vi "AK Aktion Name.vi"(11 "Aktionen":T1) -> (3 "Aktions Name":string)   [LabVIEW 2020, in "AK-Schnittstelle.lvlib"]
uses:
  AK-Schnittstelle.lvlib
  Aktionen AK.ctl
  <vilib>/Utility/Data Type/NI_Data Type.lvlib
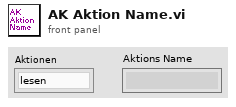
[diagram p1: front panel]
types:
  T1 = typedef "AK-Schnittstelle.lvlib/Aktionen AK.ctl" = enum16{"lesen", "initialisieren", "beenden", "AK Komm"}
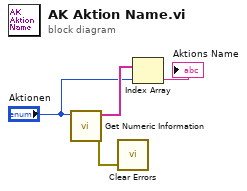
[diagram p0: block diagram]
diagram:
  n1 = call <vilib>:"Get Numeric Information.vi"("variant"="Aktionen") -> ("error out"=w4:errorcluster, "enum names"=w3:string[])  [unwired: 7 in, 2 out]
  n2 = call <vilib>:"Clear Errors.vi"("error in (no error)"=w4) -> ()  [unwired: 5 in, 2 out]
  n3 = Index Array(array=w3, index="Aktionen") -> (element=→"Aktions Name":string)
